vi "peakFinding estimateBL.vi"(5 "method":T1=1 items=["Least Square", "Least Absolute Residual", "Bisquare"], 7 "polynomial order":i32=-1, 11 "sourceData":cluster{"xData":dbl[], "yData":dbl[]}) -> (3 "estimateData":dbl[](array[numeric]), 4 "residues":dbl[](array[numeric]))   [LabVIEW 2018]
uses:
  <vilib>/Analysis/6fits.llb/Curve Fitting Criteria.ctl
  <vilib>/Analysis/NI_AALPro.lvlib
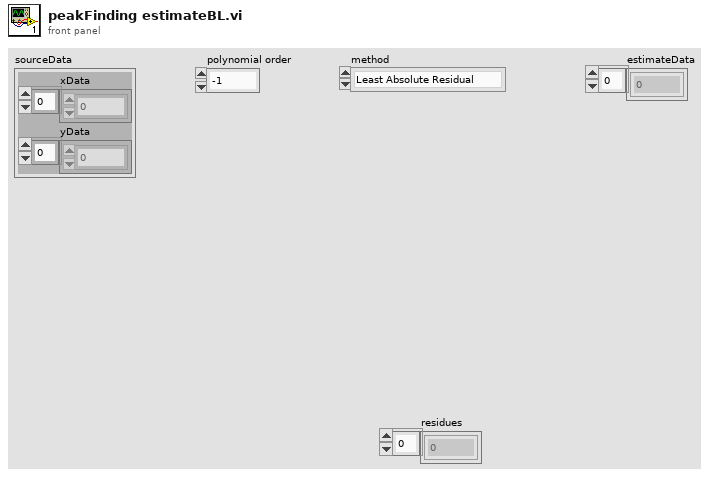
[diagram p1: front panel]
types:
  T1 = typedef "NI_AALPro.lvlib/Curve Fitting Criteria.ctl" = u16
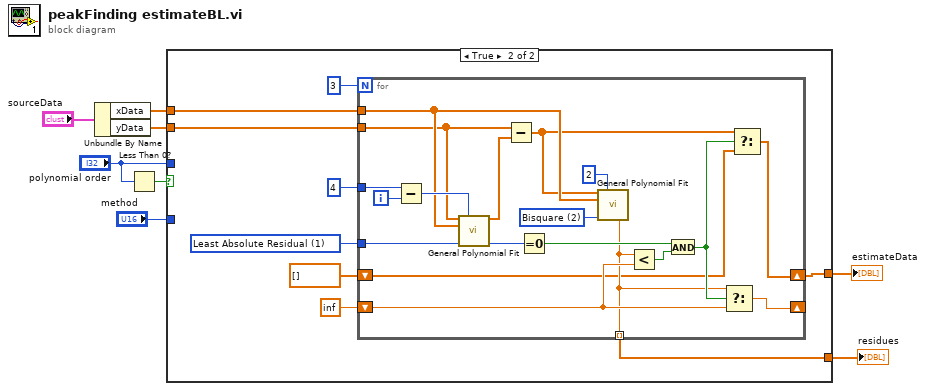
[diagram p0: block diagram]
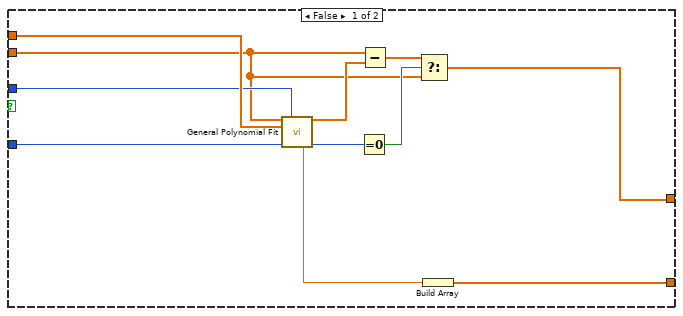
[diagram p2: hidden frame]
diagram:
  n1 = Unbundle By Name("sourceData") -> ("xData"=w6:dbl[], "yData"=w8:dbl[])
  n2 = Less Than 0?(x="polynomial order") -> (x < 0?=w4:bool)
  n3 = case shown="True" w4 {
    tunnel: w8 -> [w12 w28]
    tunnel: "method" -> [w17 _]
    tunnel: w6 -> [w19 w27]
    tunnel: "polynomial order" -> [w18 _]
    tunnel: [w11 w25] -> w2
    tunnel: [w9 w20] -> w1
    frame False {
      n4 = call <vilib>:"General Polynomial Fit.vi"("Y"=w12, "polynomial order"=w18, "X"=w19, "method"=w17) -> ("Best Polynomial Fit"=w16:dbl[], "residue"=w10:dbl, "error"=w15:i32)  [unwired: 8 in, 1 out]
      n5 = Equal To 0?(x=w15) -> (x = 0?=w14:bool)
      n6 = Subtract(x=w12, y=w16) -> (x-y=w13:dbl[])
      n7 = Select(t=w13, s=w14, f=w12) -> (s? t:f=w11:dbl[])
      n8 = Build Array(w10) -> (w9:dbl[])
    }
    frame True {
      w21 = T1 1 items=["Least Square", "Least Absolute Residual", "Bisquare"] ("method")
      n9 = for {
        N: 3 -> [_]
        tunnel: w28 -> [w32]
        tunnel: w21 -> [w47]
        tunnel: w27 -> [w44]
        tunnel: 4 -> [w41]
        shift-right: [w34] -> w25
        shift-left: dbl[] [] -> [w29]
        shift-right: [w39] -> _
        shift-left: inf ("residue") -> [w40]
        tunnel: [w31] -> w20 mode=indexing
        i -> [w46]
        w42 = T1 2 items=["Least Square", "Least Absolute Residual", "Bisquare"] ("method")
        n10 = Subtract(x=w41, y=w46) -> (x-y=w45:i32)
        n11 = call <vilib>:"General Polynomial Fit.vi"("Y"=w32, "polynomial order"=w45, "X"=w44, "method"=w47) -> ("Best Polynomial Fit"=w33:dbl[], "error"=w38:i32)  [unwired: 8 in, 2 out]
        n12 = Subtract(x=w32, y=w33) -> (x-y=w30:dbl[])
        n13 = Equal To 0?(x=w38) -> (x = 0?=w37:bool)
        n14 = call <vilib>:"General Polynomial Fit.vi"("Y"=w30, "polynomial order"=2, "X"=w44, "method"=w42) -> ("residue"=w31:dbl)  [unwired: 8 in, 3 out]
        n15 = Less?(x=w31, y=w40) -> (x < y?=w36:bool)
        n16 = And(x=w37, y=w36) -> (x .and. y?=w35:bool)
        n17 = Select(t=w31, s=w35, f=w40) -> (s? t:f=w39:dbl)
        n18 = Select(t=w30, s=w35, f=w29) -> (s? t:f=w34:dbl[])
      }
    }
  }
  "estimateData" <- w2
  "residues" <- w1
